vi "ReturnKeyPress.vi"(8 "error in (no error)":errorcluster, 11 "View in":refnum<class "View.lvclass">) -> (0 "error out":errorcluster, 3 "View out":refnum<class "View.lvclass">)   [LabVIEW 2024, in "GUI.lvlib" / "View.lvclass"]
uses:
  View.lvclass
  View.lvclass/View.ctl
  Buttons/ButtonBlack.ctl
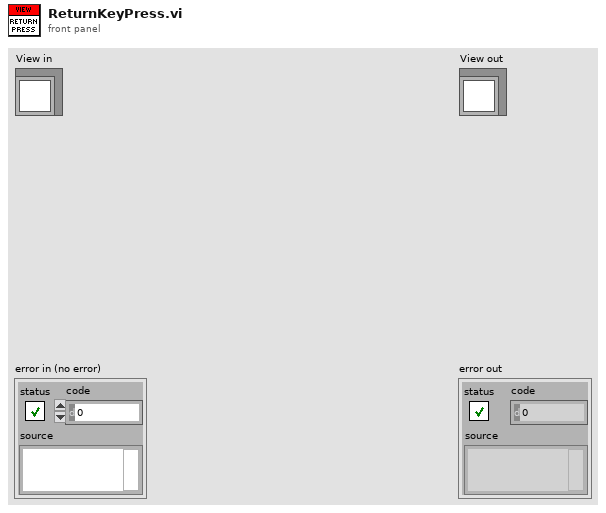
[diagram p1: front panel]
types:
  T1 = typedef "ButtonBlack.ctl" = bool
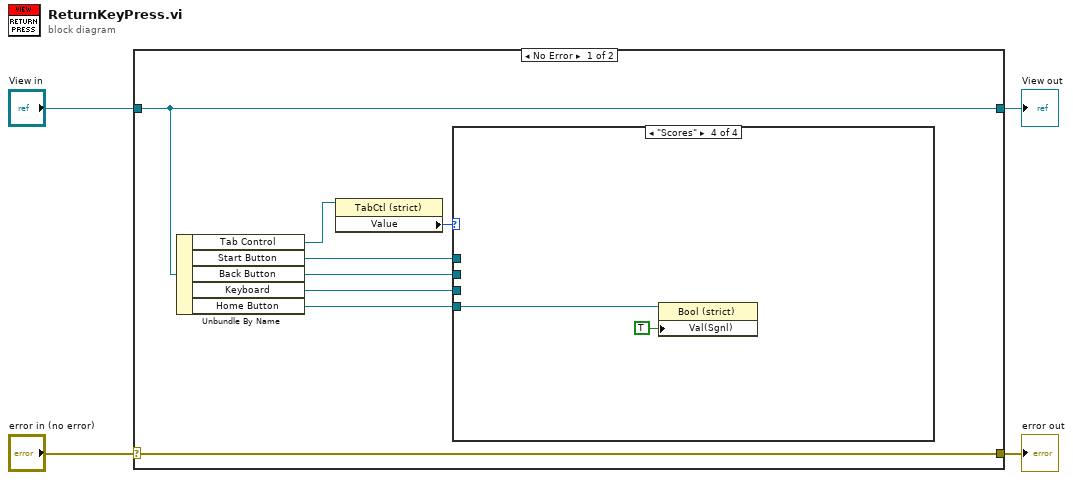
[diagram p0: block diagram]
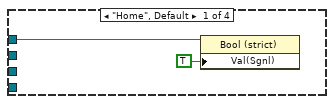
[diagram p2: hidden frame]
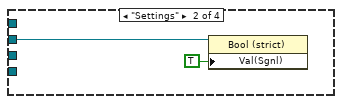
[diagram p3: hidden frame]
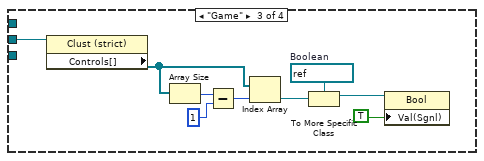
[diagram p4: hidden frame]
diagram:
  n1 = case shown="No Error" "error in (no error)" {
    selector: "error in (no error)" -> [w12 w29]
    tunnel: [w12 w29] -> w3
    tunnel: [w10 w28] -> w1
    tunnel: "View in" -> [w10 w28]
    frame No Error {
      n2 = Unbundle By Name(w10) -> ("Tab Control"=w9:refnum<vi>, "Start Button"=w7:refnum<vi>, "Back Button"=w6:refnum<vi>, "Keyboard"=w11:refnum<vi>, "Home Button"=w5:refnum<vi>)
      n3 = property class="TabCtl (strict)"(reference=w9) -> ("Value"=w8:enum32{"Home", "Settings", "Game", "Scores"})  [unwired: 1 in, 2 out]
      n4 = case shown="\"Scores\"" w8 {
        tunnel: w11 -> [_ _ w25 _]
        tunnel: w7 -> [w14 _ _ _]
        tunnel: w6 -> [_ w15 _ _]
        tunnel: w5 -> [_ _ _ w26]
        frame "Home", Default {
          n5 = property class="Bool (strict)"(reference=w14, "Val(Sgnl)"=T1 TRUE ("Value (Signaling)")) -> ()  [unwired: 1 in, 2 out]
        }
        frame "Settings" {
          n6 = property class="Bool (strict)"(reference=w15, "Val(Sgnl)"=T1 TRUE ("Value (Signaling)")) -> ()  [unwired: 1 in, 2 out]
        }
        frame "Game" {
          w22 = refnum<vi> refnum  # Boolean
          n7 = property class="Clust (strict)"(reference=w25) -> ("Controls[]"=w18:refnum<vi>[])  [unwired: 1 in, 2 out]
          n8 = Array Size(array=w18) -> (size(s)=w20:i32)
          n9 = Subtract(x=w20, y=1 ("index")) -> (x-y=w17:i32)
          n10 = Index Array(array=w18, index=w17) -> (element=w24:refnum<vi>)
          n11 = To More Specific Class(target class=w22, reference=w24) -> (specific class reference=w23:refnum<vi>)  [unwired: 1 in, 1 out]
          n12 = property class="Bool"(reference=w23, "Val(Sgnl)"=TRUE) -> ()  [unwired: 1 in, 2 out]
        }
        frame "Scores" {
          n13 = property class="Bool (strict)"(reference=w26, "Val(Sgnl)"=T1 TRUE ("Value (Signaling)")) -> ()  [unwired: 1 in, 2 out]
        }
      }
    }
    frame Error {
    }
  }
  "error out" <- w3
  "View out" <- w1
